vi "DataAnalyzer.vi"() -> ()   [LabVIEW 2014]
uses:
  <vilib>/Utility/file.llb/Read From Spreadsheet File (DBL).vi
panel:
  out "Waveform Graph 2":dbl[](graph)
  out "Waveform Graph":dbl[](graph)
  in  "Path 2":path=path "C:/Users/gplunk19/Desktop/week6/GainData.txt"
  in  "Path 3":path=path "C:/Users/gplunk19/Desktop/week6/GainData.txt"
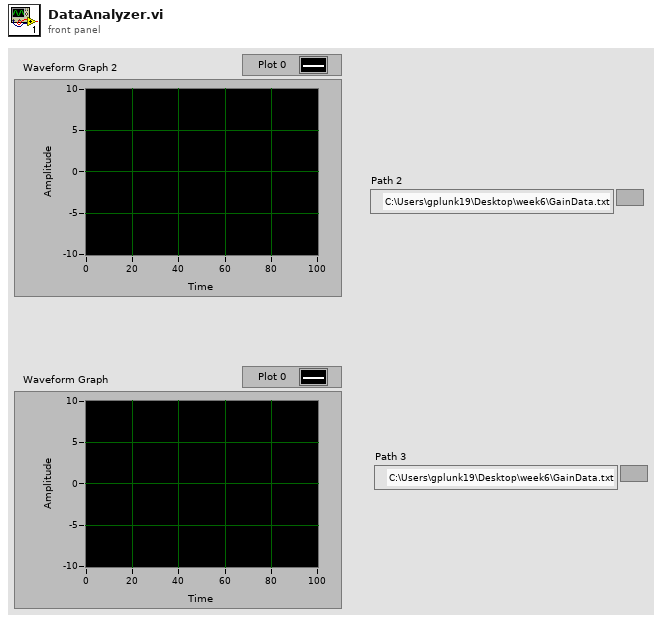
[diagram p1: front panel]
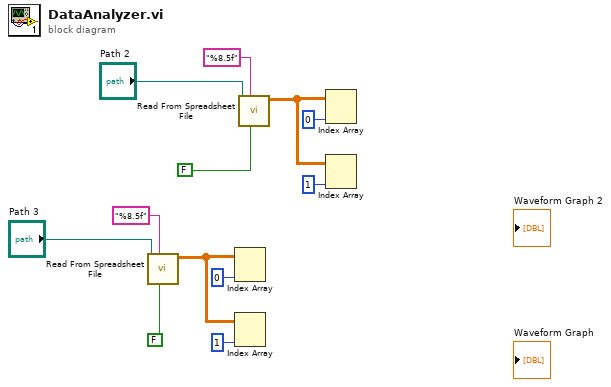
[diagram p0: block diagram]
diagram:
  n1 = call-poly <vilib>:"Read From Spreadsheet File.vi"("transpose (no:F)"=FALSE, "format (%.3f)"="%8.5f", "file path (dialog if empty)"="Path 3") -> ("all rows"=w10:dbl[][])  [unwired: 4 in, 4 out]
  n2 = Index Array(array=w10, index (col)=0) -> ()  [unwired: 1 in, 1 out]
  n3 = Index Array(array=w10, index (col)=1) -> ()  [unwired: 1 in, 1 out]
  n4 = call-poly <vilib>:"Read From Spreadsheet File.vi"("transpose (no:F)"=FALSE, "format (%.3f)"="%8.5f", "file path (dialog if empty)"="Path 2") -> ("all rows"=w4:dbl[][])  [unwired: 4 in, 4 out]
  n5 = Index Array(array=w4, index (col)=0) -> ()  [unwired: 1 in, 1 out]
  n6 = Index Array(array=w4, index (col)=1) -> ()  [unwired: 1 in, 1 out]
